vi "lvBuild.vi"() -> ()   [LabVIEW 2016, in "lvcommonbuild.lvlib"]
uses:
  lvcommonbuild.lvlib
  <vilib>/Utility/error.llb/DialogType.ctl
  <vilib>/AppBuilder/AB_API_Simple/Build (path).vi
  <vilib>/Wiresmith Technology/LabVIEW CLI/CLI Class/CLI.lvclass
  <vilib>/AppBuilder/AB_API_Simple/NI_App_Builder_API.lvlib
panel:
  out "error out":errorcluster
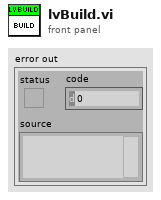
[diagram p1: front panel]
types:
  T1 = typedef "DialogType.ctl" = u16
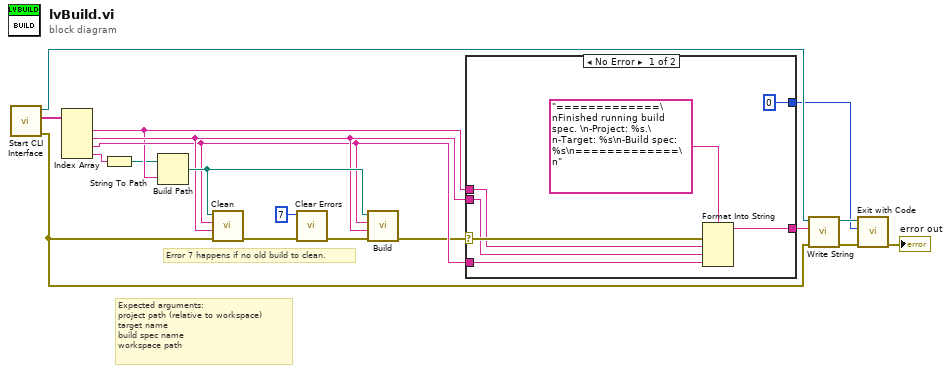
[diagram p0: block diagram]
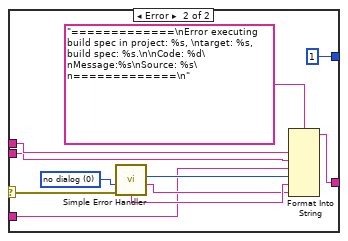
[diagram p2: hidden frame]
diagram:
  # "Error 7 happens if no old build to clean."
  # "Expected arguments:\nproject path (relative to workspace)\ntarget name\nbuild spec name\nworkspace path"
  n1 = call <vilib>:"Start CLI Interface.vi"() -> ("error out"=w7:errorcluster, "Custom Parameters"=w18:string[], "CLI out"=w16:refnum<class "CLI.lvclass">)  [unwired: 9 in]
  n2 = Index Array(array=w18) -> (element #1=w6:string, element #2=w9:string, element #3=w8:string, element #4=w1:string)  [unwired: 4 in]
  n3 = String To Path(string=w1) -> (path=w5:path)
  n4 = Build Path(base path=w5, name or relative path=w6) -> (appended path=w10:path)
  n5 = call <vilib>:"Clean.vi"("error in (no error)"=w7, "Name of target (My Computer)"=w9, "Name of build specification (if empty: clean all)"=w8, "Path to project"=w10) -> ("error out"=w11:errorcluster)  [unwired: 7 in]
  n6 = call <vilib>:"Clear Errors.vi"("error in (no error)"=w11, "specific error code to clear (0: all)"=7) -> ("error out"=w4:errorcluster)  [unwired: 4 in, 1 out]
  n7 = call-poly <vilib>:"Build.vi"("error in (no error)"=w4, "Name of target (My Computer)"=w9, "Name of build specification (if empty: build all)"=w8, "Path to project"=w10) -> ("error out"=w2:errorcluster)  [unwired: 6 in, 1 out]
  n8 = case shown="No Error" w2 {
    selector: w2 -> [w24 w35]
    tunnel: w6 -> [w23 w28]
    tunnel: w9 -> [w22 w27]
    tunnel: [w21 w36] -> w17
    tunnel: [0 ("Exit Code (0)") 1 ("Exit Code (0)")] -> w13
    tunnel: w8 -> [w19 w26]
    frame No Error {
      n9 = Format Into String(format string="=============\nFinished running build spec. \n-Project: %s.\n-Target: %s\n-Build spec: %s\n=============\n", error in=w24, w23, w22, w19) -> (resulting string=w21:string)  [unwired: 1 in, 1 out]
    }
    frame Error {
      w34 = T1 0 items=["no dialog", "OK message", "continue or stop message", "OK message + warnings", "continue/stop + warnings"] ("type of dialog (OK msg:1)")
      n10 = call <vilib>:"Simple Error Handler.vi"("type of dialog (OK msg:1)"=w34, "error in (no error)"=w35) -> ("code out"=w29:i32, "source out"=w30:string, "message"=w31:string)  [unwired: 3 in, 2 out]
      n11 = Format Into String(format string="=============\nError executing build spec in project: %s, \ntarget: %s, build spec: %s.\n\nCode: %d\nMessage:%s\nSource: %s\n=============\n", w28, w27, w26, w29, w31, w30) -> (resulting string=w36:string)  [unwired: 2 in, 1 out]
    }
  }
  n12 = call <vilib>:"Write String.vi"("error in (no error)"=w7, "Text to Write"=w17, "CLI in"=w16) -> ("error out"=w15:errorcluster, "CLI out"=w14:refnum<class "CLI.lvclass">)  [unwired: 7 in]
  n13 = call <vilib>:"Exit with Code.vi"("error in (no error)"=w15, "Exit Code (0)"=w13, "CLI in"=w14) -> ("error out"=→"error out":errorcluster)  [unwired: 8 in]
